vi "SDO Download__.vi"(6 "Data":variant, 7 "Wait?":bool, 8 "error in":errorcluster, 9 "Multiplexer":T1 {"Sub-Index" format="%.0x"; "Index" format="%.0x"}, 10 "Node ID":u8, 11 "CANopen in":refnum<class "CANopen.lvclass">) -> (0 "error out":errorcluster, 3 "CANopen out":refnum<class "CANopen.lvclass">)   [LabVIEW 2024, in "CANopen.lvlib" / "CANopen.lvclass"]
doc: "Write value into remote device's object dictionary."
uses:
  CANopen.lvclass
  CANopen.lvclass/CANopen.ctl
  COB Peer-To-Peer.ctl
  Multiplexer.ctl
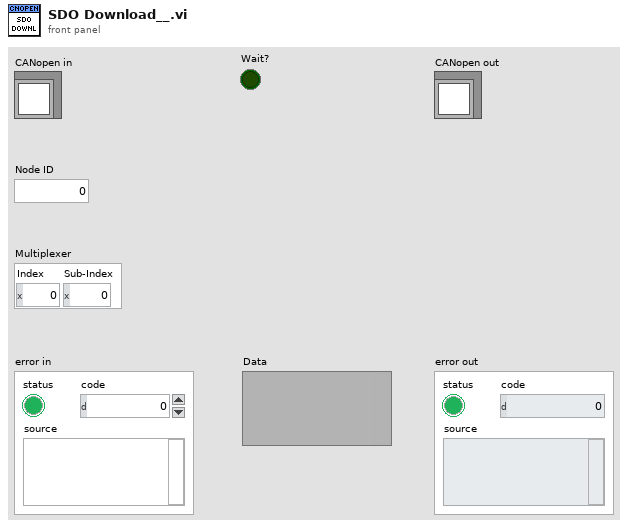
[diagram p1: front panel]
types:
  T1 = typedef "canopen.lvlib/CANopen.lvclass/Multiplexer.ctl" = cluster{"Index":u16, "Sub-Index":u8}
  T2 = typedef "COB Peer-To-Peer.ctl" = u16
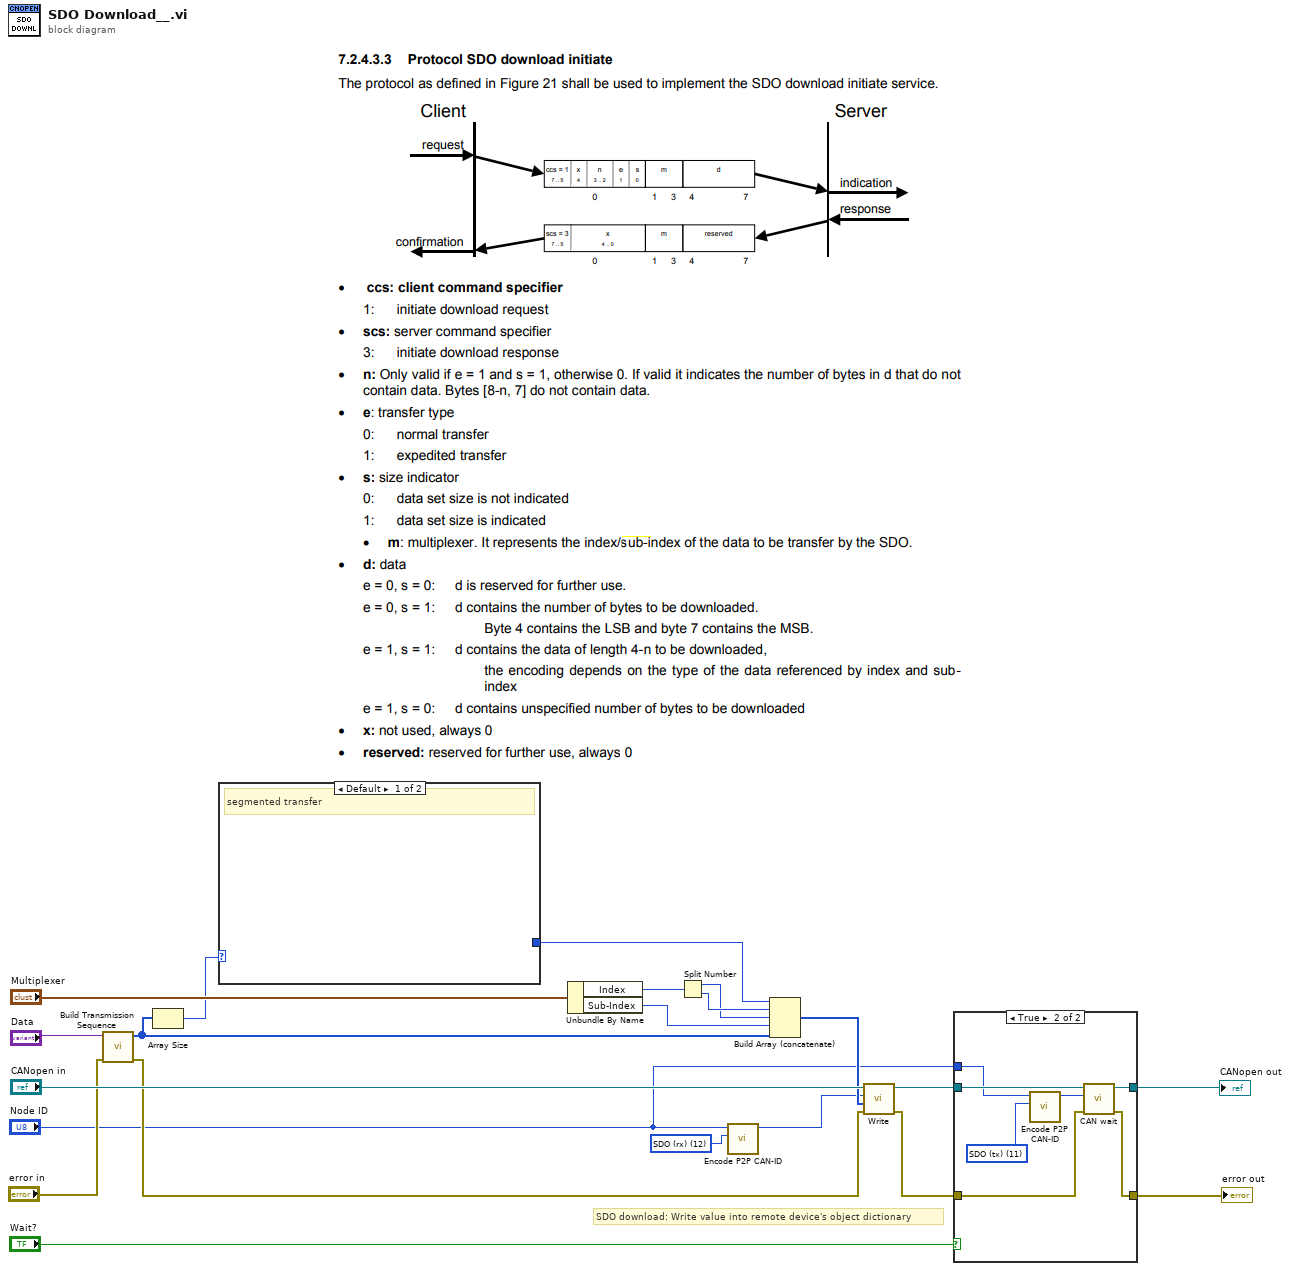
[diagram p0: block diagram]
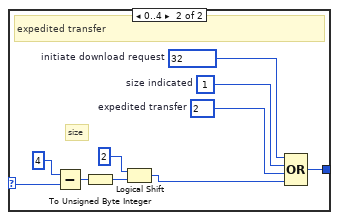
[diagram p3: hidden frame]
diagram:
  w8 = T2 12 items=["EMCY"=1, "PDO1 (tx)"=3, "PDO1 (rx)"=4, "PDO2 (tx)"=5, "PDO2 (rx)"=6, "PDO3 (tx)"=7, "PDO3 (rx)"=8, "PDO4 (tx)"=9, "PDO4 (rx)"=10, "SDO (tx)"=11, "SDO (rx)"=12, "NMT error control"=14] ("COB Peer-To-Peer")
  # "SDO download: Write value into remote device's object dictionary"
  n1 = call "Build Transmission Sequence.vi"("error in"="error in", "Data"="Data") -> ("error out"=w12:errorcluster, "Transmission Sequence"=w11:u8[])  [unwired: 8 in]
  n2 = Array Size(array=w11) -> (size(s)=w10:i32)
  n3 = case shown="Default" w10 {
    selector: w10 -> [_ w26]
    tunnel: [_ w28] -> w9
    frame Default {
      # "segmented transfer"
    }
    frame 0..4 {
      w29 = u8 2  # expedited transfer
      w30 = u8 1  # size indicated
      w31 = u8 32  # initiate download request
      # "size"
      # "expedited transfer"
      n4 = Subtract(x=4 ("y"), y=w26) -> (x-y=w25:i32)
      n5 = To Unsigned Byte Integer(number=w25) -> (unsigned 8bit integer=w24:u8)
      n6 = Logical Shift(y=i8 2, x=w24) -> (x << y=w22:u8)
      n7 = Compound Arithmetic op=OR(w31, w30, w29, w22) -> (w28:u8)
    }
  }
  n8 = Unbundle By Name("Multiplexer") -> ("Index"=w19:u16, "Sub-Index"=w16:u8)
  n9 = Split Number(x=w19) -> (hi(x)=w17:u8, lo(x)=w18:u8)
  n10 = call "Encode P2P CAN-ID.vi"("COB Peer-To-Peer"=w8, "Node ID"="Node ID") -> ("CAN-ID"=w2:u32)  [unwired: 9 in]
  n11 = Build Array (concatenate)(w9, w18, w17, w16, w11) -> (w14:u8[])
  n12 = call "Write.vi"("error in"=w12, "Data"=w14, "CAN-ID"=w2, "CANopen in"="CANopen in") -> ("error out"=w5:errorcluster, "CANopen out"=w7:refnum<class "CANopen.lvclass">)  [unwired: 6 in]
  n13 = case shown="True" "Wait?" {
    tunnel: w7 -> [w33 w40]
    tunnel: [w33 w39] -> w6
    tunnel: [w32 w38] -> w4
    tunnel: w5 -> [w32 w37]
    tunnel: "Node ID" -> [_ w35]
    frame False {
    }
    frame True {
      w34 = T2 11 items=["EMCY"=1, "PDO1 (tx)"=3, "PDO1 (rx)"=4, "PDO2 (tx)"=5, "PDO2 (rx)"=6, "PDO3 (tx)"=7, "PDO3 (rx)"=8, "PDO4 (tx)"=9, "PDO4 (rx)"=10, "SDO (tx)"=11, "SDO (rx)"=12, "NMT error control"=14] ("COB Peer-To-Peer")
      n14 = call "Encode P2P CAN-ID.vi"("COB Peer-To-Peer"=w34, "Node ID"=w35) -> ("CAN-ID"=w36:u32)  [unwired: 9 in]
      n15 = call "CAN wait.vi"("error in (no error)"=w37, "Cob ID"=w36, "CANopen in"=w40) -> ("error out"=w38:errorcluster, "CANopen out"=w39:refnum<class "CANopen.lvclass">)  [unwired: 1 in, 2 out]
    }
  }
  "CANopen out" <- w6
  "error out" <- w4
